vi "Func-Math-Finder-03022016.vi"(4 "All Fn-Math":string[](array[string]), 6 "All Fn Name":string[](array[string]), 7 "Func Name":string, 8 "error in (no error)":errorcluster, 11 "Get Tagged String":string) -> (0 "error out":errorcluster, 1 "is empty?":string, 2 "Expression":string)   [LabVIEW 2014]
doc: "This VI takes tagged string from SBML parser.vi as input and translate it into kinetic law. It supports the following five mathematical functions:\n+, -, *, /, pow\n\nDesigned by HB\nhaba@dtu.dk"
uses:
  <vilib>/regexp/Match Regular Expression.xnode
panel:
  out "RHS ex":string
  out "Inter. exp":string
  in  "RHS":string
  in  "LHS":string
  # "multiplySOP1k1, addSOP2S1, S2EOP2, subSOP2k1, 4EOP2EOP1"
  # "SOP1 + x 2 EOP1"
  # "SOP1 + SOP2 * a b EOP2 c EOP1"
  # "SOP1 + c SOP2 * a b EOP2 EOP1"
  # "SOP1 + SOP2 * a SOP3 pow x 2 EOP3 EOP2 SOP2 * b x EOP2 c EOP1"
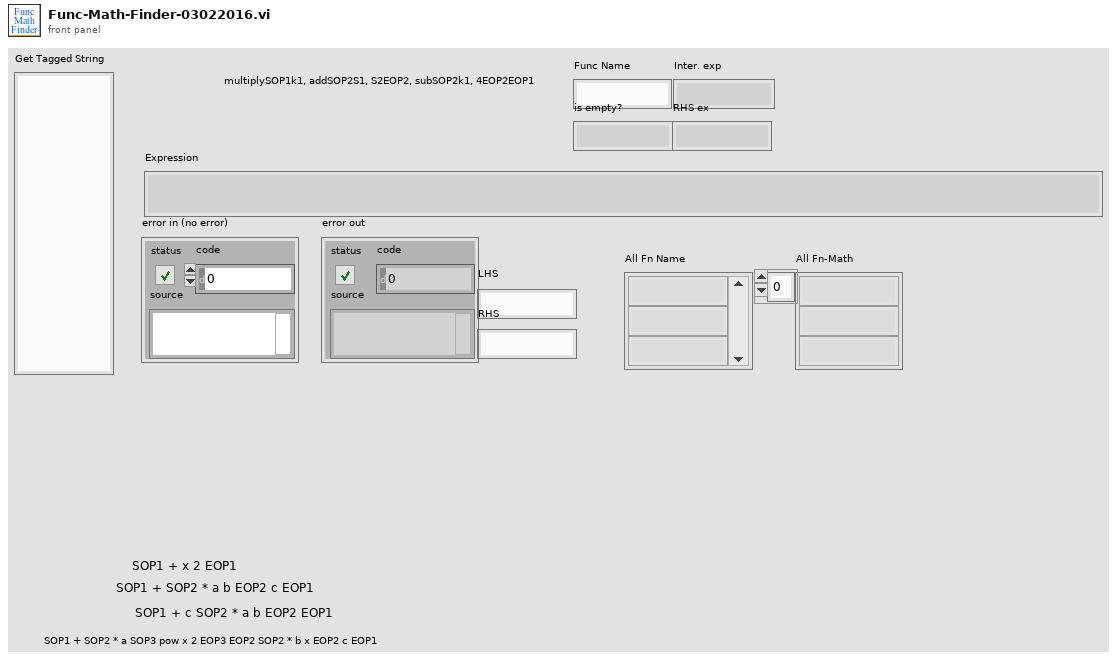
[diagram p1: front panel]
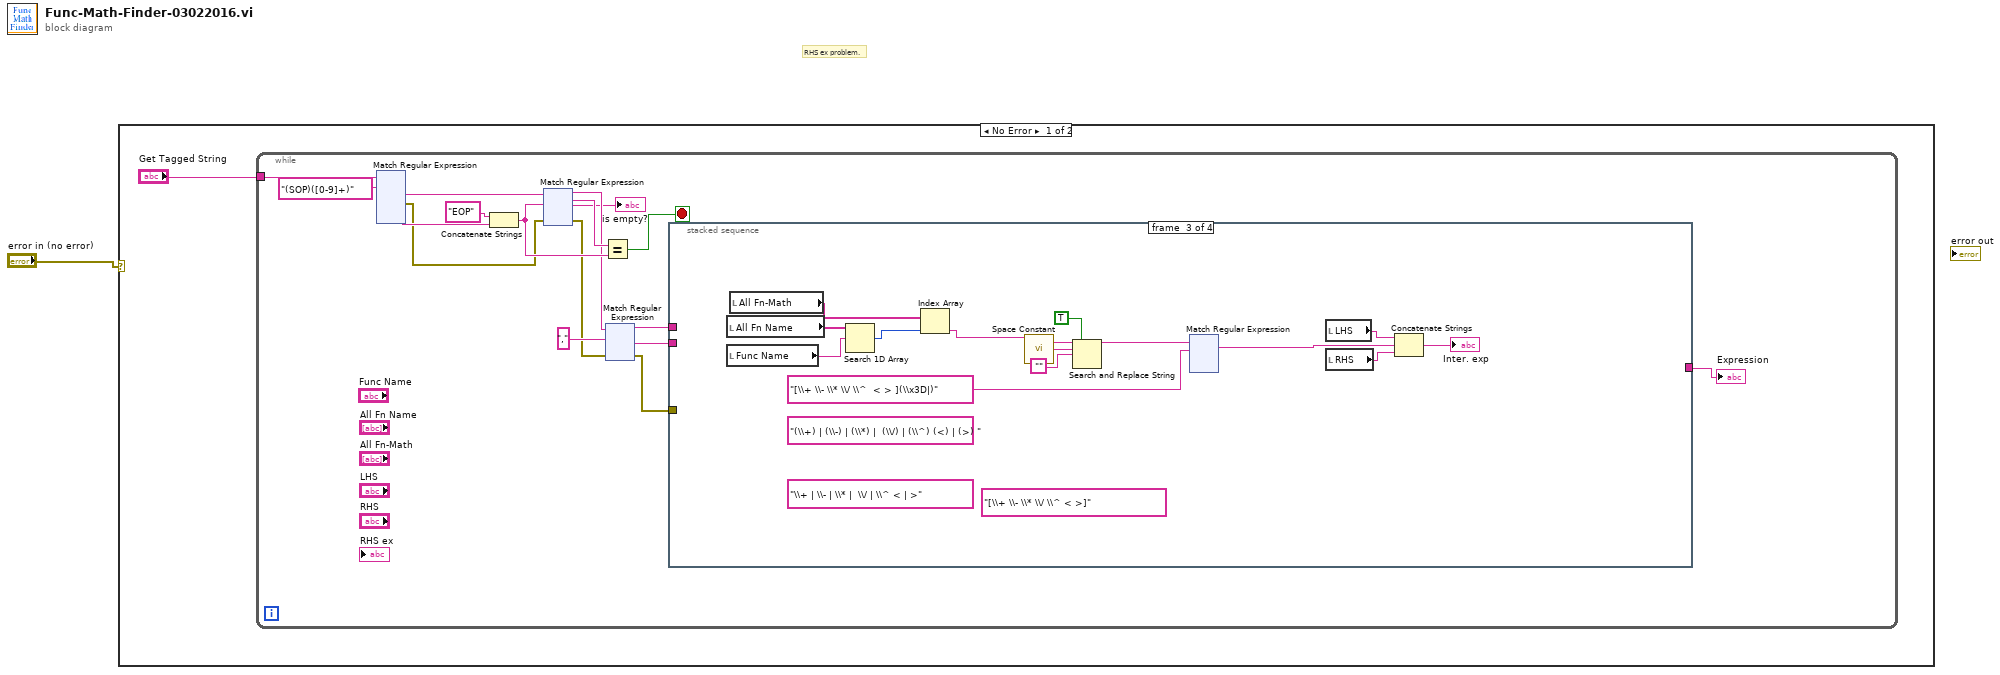
[diagram p0: block diagram]
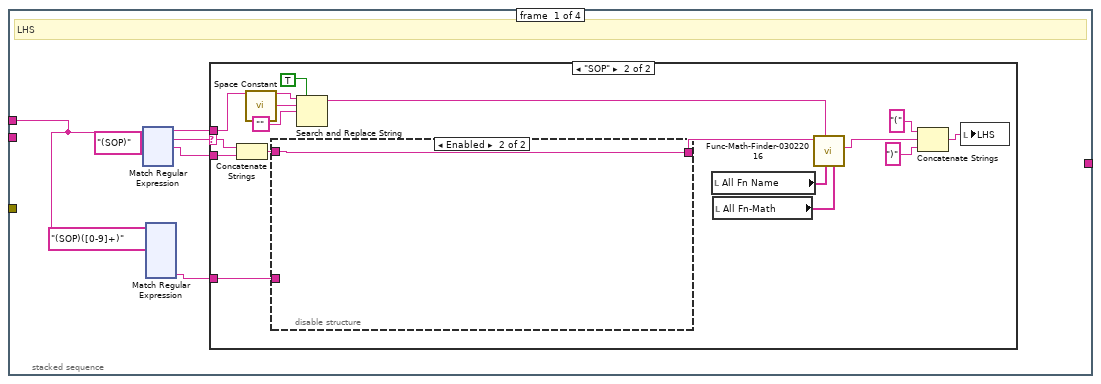
[diagram p2: hidden frame]
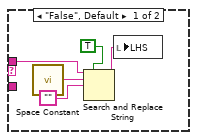
[diagram p3: hidden frame]
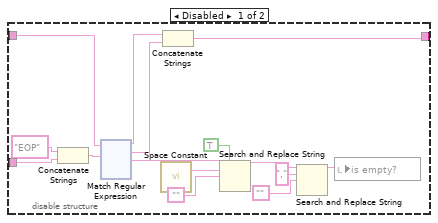
[diagram p4: hidden frame]
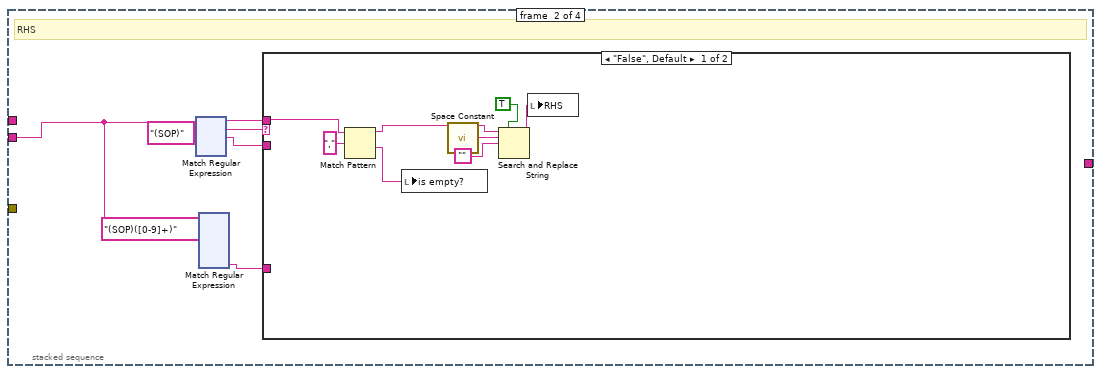
[diagram p5: hidden frame]
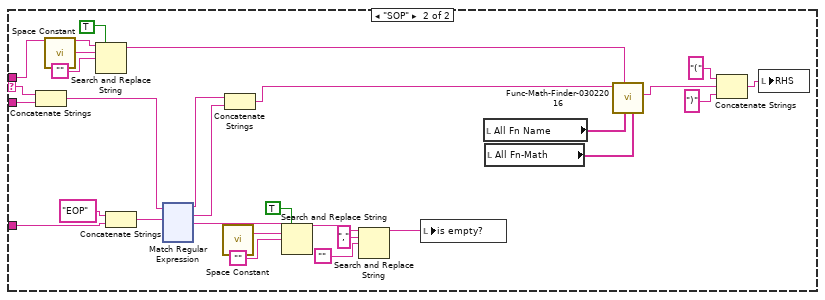
[diagram p6: hidden frame]
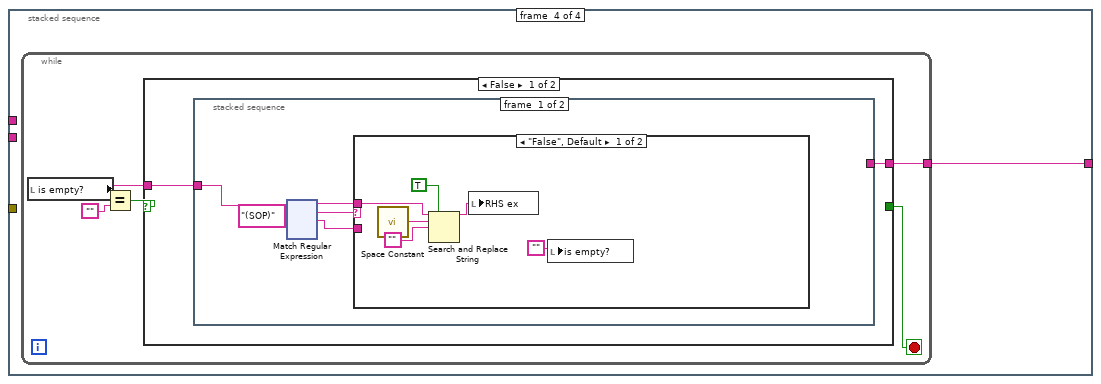
[diagram p7: hidden frame]
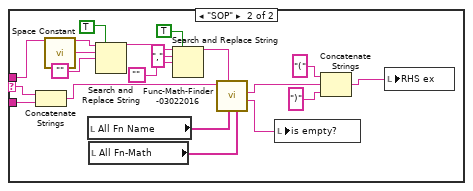
[diagram p8: hidden frame]
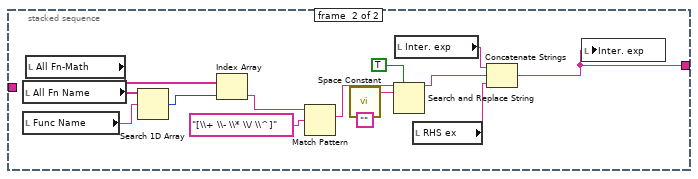
[diagram p9: hidden frame]
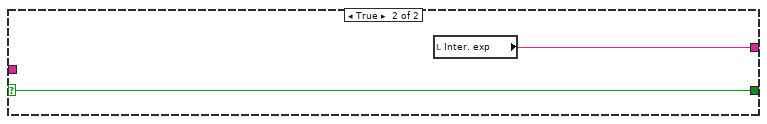
[diagram p10: hidden frame]
diagram:
  # "RHS ex problem."
  n1 = case shown="No Error" "error in (no error)" {
    frame No Error {
      n2 = while {
        tunnel: "Get Tagged String" -> [w10]
        stop <- w17 stop-if-true
        n3 = xnode "Match Regular Expression"("input string"=w10, "regular expression"="(SOP)([0-9]+)") -> ("after match"=w13:string, "error out"=w9:errorcluster, "submatch 2"=w12:string)  [unwired: 4 in, 4 out]
        n4 = Concatenate Strings("EOP" ("regular expression"), w12) -> (w18:string)
        n5 = xnode "Match Regular Expression"("input string"=w13, "regular expression"=w18, "error in"=w9) -> ("before match"=w15:string, "whole match"=w16:string, "after match"=→"is empty?":string, "error out"=w8:errorcluster)  [unwired: 3 in, 1 out]
        n6 = Equal?(x=w16, y=w18) -> (x = y?=w17:bool)
        n7 = xnode "Match Regular Expression"("input string"=w15, "regular expression"="," ("Oprts Lst"), "error in"=w8) -> ("before match"=w7:string, "after match"=w5:string, "error out"=w6:errorcluster)  [unwired: 3 in, 2 out]
        n8 = stacked-sequence {
          tunnel: w7 -> [w20 _ _ _]
          tunnel: w6 -> [_ _ _ _]
          tunnel: w5 -> [_ w410 _ _]
          tunnel: [_ _ _ w925] -> w4
          frame #0 {
            # "LHS"
            n9 = xnode "Match Regular Expression"("input string"=w20, "regular expression"="(SOP)") -> ("before match"=w23:string, "whole match"=w25:string, "after match"=w24:string)  [unwired: 4 in, 2 out]
            n10 = xnode "Match Regular Expression"("input string"=w20, "regular expression"="(SOP)([0-9]+)") -> ("submatch 2"=w21:string)  [unwired: 4 in, 6 out]
            n11 = case shown="\"SOP\"" w25 {
              selector: w25 -> [_ w164]
              tunnel: w23 -> [w145 w155]
              tunnel: w24 -> [_ w163]
              tunnel: w21 -> [_ w151]
              frame "False", Default {
                n12 = call <vilib>:"Space Constant.vi"() -> ("String"=w147:string)
                n13 = Search and Replace String(replace all?=TRUE ("replace all? (F)"), input string=w145, search string=w147, replace string="" ("string")) -> (result string=w144:string)  [unwired: 4 in, 3 out]
                n14 = local write "LHS"(w144) -> ()
              }
              frame "SOP" {
                n15 = Concatenate Strings(w164, w163) -> (w150:string)
                n16 = call <vilib>:"Space Constant.vi"() -> ("String"=w156:string)
                n17 = disable-structure shown="Enabled" {
                  disable-tunnel: w151 -> [w178 _]
                  disable-tunnel: w150 -> [w168 w294]
                  disable-tunnel: [w167 w294] -> w149
                  frame Disabled {
                    n18 = Concatenate Strings("EOP" ("regular expression"), w178) -> (w177:string)
                    n19 = xnode "Match Regular Expression"("input string"=w168, "regular expression"=w177) -> ("before match"=w169:string, "whole match"=w170:string, "after match"=w172:string)  [unwired: 4 in, 2 out]
                    n20 = call <vilib>:"Space Constant.vi"() -> ("String"=w175:string)
                    n21 = Concatenate Strings(w169, w170) -> (w167:string)
                    n22 = Search and Replace String(replace all?=TRUE ("replace all? (F)"), input string=w172, search string=w175, replace string="" ("string")) -> (result string=w174:string)  [unwired: 4 in, 3 out]
                    n23 = Search and Replace String(input string=w174, search string=",", replace string="" ("string")) -> (result string=w171:string)  [unwired: 5 in, 3 out]
                    n24 = local write "is empty?"(w171) -> ()
                  }
                  frame Enabled {
                  }
                }
                n25 = Search and Replace String(replace all?=TRUE ("replace all? (F)"), input string=w155, search string=w156, replace string="" ("string")) -> (result string=w154:string)  [unwired: 4 in, 3 out]
                n26 = local read "All Fn Name"() -> (w153:string[])
                n27 = local read "All Fn-Math"() -> (w152:string[])
                n28 = call "Func-Math-Finder-03022016.vi"("All Fn-Math"=w152, "All Fn Name"=w153, "Func Name"=w154, "Get Tagged String"=w149) -> ("Expression"=w159:string)  [unwired: 5 in, 2 out]
                n29 = Concatenate Strings("(" ("string"), w159, ")" ("string")) -> (w160:string)
                n30 = local write "LHS"(w160) -> ()
              }
            }
          }
          frame #1 {
            # "RHS"
            n31 = xnode "Match Regular Expression"("input string"=w410, "regular expression"="(SOP)") -> ("before match"=w412:string, "whole match"=w414:string, "after match"=w413:string)  [unwired: 4 in, 2 out]
            n32 = xnode "Match Regular Expression"("input string"=w410, "regular expression"="(SOP)([0-9]+)") -> ("submatch 2"=w409:string)  [unwired: 4 in, 6 out]
            n33 = case shown="\"False\", Default" w414 {
              selector: w414 -> [_ w568]
              tunnel: w412 -> [w536 w559]
              tunnel: w413 -> [_ w567]
              tunnel: w409 -> [_ w554]
              frame "False", Default {
                n34 = Match Pattern(string=w536, regular expression=",") -> (before substring=w534:string, after substring=w533:string)  [unwired: 1 in, 2 out]
                n35 = local write "is empty?"(w533) -> ()
                n36 = call <vilib>:"Space Constant.vi"() -> ("String"=w539:string)
                n37 = Search and Replace String(replace all?=TRUE ("replace all? (F)"), input string=w534, search string=w539, replace string="" ("string")) -> (result string=w537:string)  [unwired: 4 in, 3 out]
                n38 = local write "RHS"(w537) -> ()
              }
              frame "SOP" {
                n39 = Concatenate Strings(w568, w567) -> (w544:string)
                n40 = call <vilib>:"Space Constant.vi"() -> ("String"=w560:string)
                n41 = Search and Replace String(replace all?=TRUE ("replace all? (F)"), input string=w559, search string=w560, replace string="" ("string")) -> (result string=w558:string)  [unwired: 4 in, 3 out]
                n42 = Concatenate Strings("EOP" ("regular expression"), w554) -> (w553:string)
                n43 = xnode "Match Regular Expression"("input string"=w544, "regular expression"=w553) -> ("before match"=w545:string, "whole match"=w546:string, "after match"=w548:string)  [unwired: 4 in, 2 out]
                n44 = call <vilib>:"Space Constant.vi"() -> ("String"=w551:string)
                n45 = Concatenate Strings(w545, w546) -> (w543:string)
                n46 = Search and Replace String(replace all?=TRUE ("replace all? (F)"), input string=w548, search string=w551, replace string="" ("string")) -> (result string=w550:string)  [unwired: 4 in, 3 out]
                n47 = Search and Replace String(input string=w550, search string=",", replace string="" ("string")) -> (result string=w547:string)  [unwired: 5 in, 3 out]
                n48 = local write "is empty?"(w547) -> ()
                n49 = local read "All Fn Name"() -> (w557:string[])
                n50 = local read "All Fn-Math"() -> (w556:string[])
                n51 = call "Func-Math-Finder-03022016.vi"("All Fn-Math"=w556, "All Fn Name"=w557, "Func Name"=w558, "Get Tagged String"=w543) -> ("Expression"=w563:string)  [unwired: 5 in, 2 out]
                n52 = Concatenate Strings("(" ("string"), w563, ")" ("string")) -> (w564:string)
                n53 = local write "RHS"(w564) -> ()
              }
            }
          }
          frame #2 {
            (unwired) "[\\+ \\- \\* \\/ \\^ < >]" ("Oprts Lst")
            (unwired) "\\+ | \\- | \\* |  \\/ | \\^ < | >" ("Oprts Lst")
            (unwired) "(\\+) | (\\-) | (\\*) |  (\\/) | (\\^) (<) | (>) " ("Oprts Lst")
            n54 = local read "All Fn Name"() -> (w806:string[])
            n55 = local read "Func Name"() -> (w804:string)
            n56 = local read "All Fn-Math"() -> (w805:string[])
            n57 = Search 1D Array(1D array=w806, element=w804) -> (index of element=w807:i32)  [unwired: 1 in]
            n58 = Index Array(array=w805, index=w807) -> (element=w799:string)
            n59 = call <vilib>:"Space Constant.vi"() -> ("String"=w801:string)
            n60 = Search and Replace String(replace all?=TRUE ("replace all? (F)"), input string=w799, search string=w801, replace string="" ("string")) -> (result string=w797:string)  [unwired: 4 in, 3 out]
            n61 = xnode "Match Regular Expression"("input string"=w797, "regular expression"="[\\+ \\- \\* \\/ \\^  < > ](\\x3D|)" ("Oprts Lst")) -> ("whole match"=w798:string)  [unwired: 4 in, 4 out]
            n62 = local read "LHS"() -> (w810:string)
            n63 = local read "RHS"() -> (w809:string)
            n64 = Concatenate Strings(w810, w798, w809) -> (→"Inter. exp":string)
          }
          frame #3 {
            n65 = while {
              tunnel: [w927] -> w925
              stop <- w928 stop-if-true
              n66 = local read "is empty?"() -> (w926:string)
              n67 = Equal?(x=w926, y="") -> (x = y?=w929:bool)
              n68 = case shown="False" w929 {
                selector: w929 -> [_ w1091]
                tunnel: [_ w1091] -> w928
                tunnel: [w931 w1090] -> w927
                tunnel: w926 -> [w932 _]
                frame False {
                  n69 = stacked-sequence {
                    tunnel: w932 -> [w933 _]
                    tunnel: [_ w1084] -> w931
                    frame #0 {
                      n70 = xnode "Match Regular Expression"("input string"=w933, "regular expression"="(SOP)") -> ("before match"=w934:string, "whole match"=w936:string, "after match"=w935:string)  [unwired: 4 in, 2 out]
                      n71 = case shown="\"False\", Default" w936 {
                        selector: w936 -> [_ w962]
                        tunnel: w934 -> [w940 w952]
                        tunnel: w935 -> [_ w961]
                        frame "False", Default {
                          n72 = call <vilib>:"Space Constant.vi"() -> ("String"=w942:string)
                          n73 = Search and Replace String(replace all?=TRUE ("replace all? (F)"), input string=w940, search string=w942, replace string="" ("string")) -> (result string=w939:string)  [unwired: 4 in, 3 out]
                          n74 = local write "RHS ex"(w939) -> ()
                          n75 = local write "is empty?"("") -> ()
                        }
                        frame "SOP" {
                          n76 = Concatenate Strings(w962, w961) -> (w960:string)
                          n77 = call <vilib>:"Space Constant.vi"() -> ("String"=w953:string)
                          n78 = local read "All Fn Name"() -> (w951:string[])
                          n79 = local read "All Fn-Math"() -> (w950:string[])
                          n80 = Search and Replace String(replace all?=TRUE ("replace all? (F)"), input string=w952, search string=w953, replace string="" ("string")) -> (result string=w947:string)  [unwired: 4 in, 3 out]
                          n81 = Search and Replace String(replace all?=TRUE ("replace all? (F)"), input string=w947, search string=",", replace string="" ("string")) -> (result string=w945:string)  [unwired: 4 in, 3 out]
                          n82 = call "Func-Math-Finder-03022016.vi"("All Fn-Math"=w950, "All Fn Name"=w951, "Func Name"=w945, "Get Tagged String"=w960) -> ("is empty?"=w944:string, "Expression"=w956:string)  [unwired: 5 in, 1 out]
                          n83 = local write "is empty?"(w944) -> ()
                          n84 = Concatenate Strings("(" ("string"), w956, ")" ("string")) -> (w957:string)
                          n85 = local write "RHS ex"(w957) -> ()
                        }
                      }
                    }
                    frame #1 {
                      (unwired) "" ("string")
                      n86 = local read "All Fn Name"() -> (w1080:string[])
                      n87 = local read "Func Name"() -> (w1078:string)
                      n88 = local read "All Fn-Math"() -> (w1079:string[])
                      n89 = Search 1D Array(1D array=w1080, element=w1078) -> (index of element=w1082:i32)  [unwired: 1 in]
                      n90 = Index Array(array=w1079, index=w1082) -> (element=w1081:string)
                      n91 = Match Pattern(string=w1081, regular expression="[\\+ \\- \\* \\/ \\^]" ("Oprts Lst")) -> (match substring=w1077:string)  [unwired: 1 in, 3 out]
                      n92 = call <vilib>:"Space Constant.vi"() -> ("String"=w1088:string)
                      n93 = Search and Replace String(replace all?=TRUE ("replace all? (F)"), input string=w1077, search string=w1088) -> (result string=w1087:string)  [unwired: 5 in, 3 out]
                      n94 = local read "Inter. exp"() -> (w1086:string)
                      n95 = local read "RHS ex"() -> (w1085:string)
                      n96 = Concatenate Strings(w1086, w1087, w1085) -> (w1084:string)
                      n97 = local write "Inter. exp"(w1084) -> ()
                    }
                  }
                }
                frame True {
                  n98 = local read "Inter. exp"() -> (w1090:string)
                }
              }
            }
          }
        }
        "Expression" <- w4
      }
    }
    frame Error {
    }
  }
